vi "q_update_offset.vi"(1 "Q2 valid":bool=TRUE, 3 "Q1 valid":bool=TRUE, 5 "Q1_temp":fxp<+/-,32,16>, 7 "Q2_temp":fxp<+/-,32,16>, 8 "x_offset":fxp<+/-,16,8>, 10 "y_offset":fxp<+/-,16,8>) -> (15 "Q1temp_out":fxp<+/-,32,16>, 16 "q1temp_valid":bool, 18 "Q2temp_out":fxp<+/-,32,16>, 19 "q2temp_valid":bool)   [LabVIEW 2020]
uses:
  <vilib>/rvi/FXPMathLib/FxpSub/XNode/nifxpmath_Sub.xnode
  <vilib>/rvi/FXPMathLib/sim/FxpSim.dll
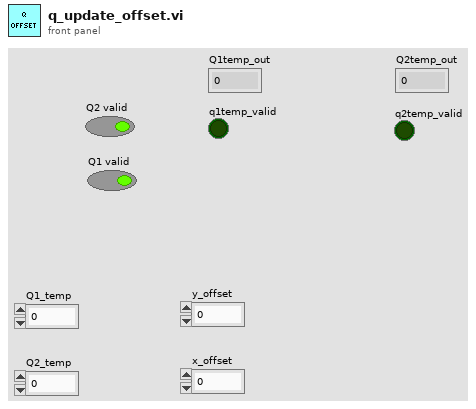
[diagram p1: front panel]
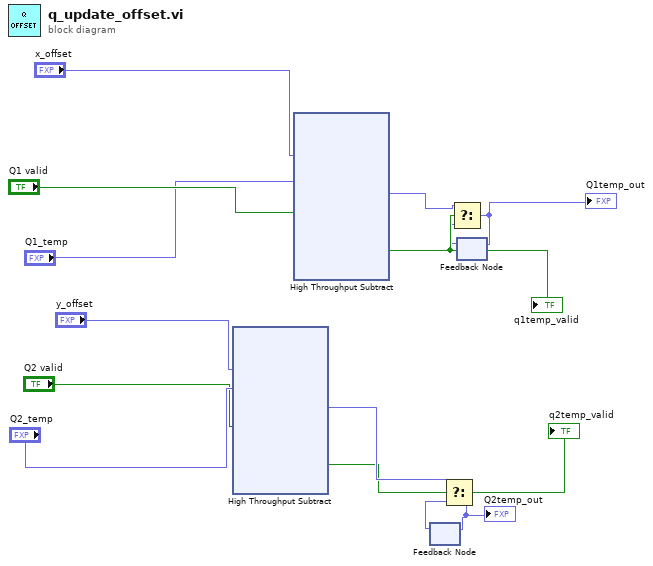
[diagram p0: block diagram]
diagram:
  n1 = xnode "High Throughput Subtract"("x"="y_offset", "y"="Q2_temp", "input valid"="Q2 valid") -> ("x-y"=w14:fxp<+/-,32,16>, "output valid"=w13:bool)  [unwired: 1 in, 1 out]
  "q2temp_valid" <- w13
  n2 = xnode "High Throughput Subtract"("x"="x_offset", "y"="Q1_temp", "input valid"="Q1 valid") -> ("x-y"=w5:fxp<+/-,32,16>, "output valid"=w7:bool)  [unwired: 1 in, 1 out]
  "q1temp_valid" <- w7
  n3 = feedback #1() -> (w12:fxp<+/-,32,16>)  [unwired: 1 in]
  n4 = Select(t=w14, s=w13, f=w12) -> (s? t:f=w2:fxp<+/-,32,16>)
  "Q2temp_out" <- w2
  n5 = feedback-in #1(w2) -> ()
  n6 = feedback #2() -> (w6:fxp<+/-,32,16>)  [unwired: 1 in]
  n7 = Select(t=w5, s=w7, f=w6) -> (s? t:f=w4:fxp<+/-,32,16>)
  "Q1temp_out" <- w4
  n8 = feedback-in #2(w4) -> ()
